vi "LOAD CELL FGV MAIN.vi"(7 "Enum":T2(ring), 8 "error in (no error)":errorcluster, 11 "main ref":T1) -> (0 "error IO":errorcluster)   [LabVIEW 2025]
uses:
  controls/LAB-IQ UI Data.ctl
  lib/hps_ft.dll
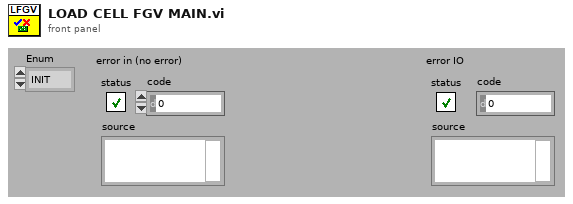
[diagram p1: front panel]
types:
  T1 = typedef "LAB-IQ UI Data.ctl" = cluster{"Main Home Screen":cluster{"GUI":refnum<vi>, "Platform Settings":refnum<vi>, "Configure":refnum<vi>, "Home":refnum<vi>, "EXIT":refnum<vi>, "service 2":refnum<vi>, "MainPage":refnum<vi>, "Analysis":refnum<vi>}, "Platform Settings":cluster{"mm/s  Surge":refnum<vi>, "Update Surge Speed":refnum<vi>, "Drive Error":refnum<vi>, "Disable Axis Jog Soft Limits":refnum<vi>, "mm/s  Sway":refnum<vi>, "Sway and Surge COM Status":refnum<vi>, "Heave COM Status":refnum<vi>, "Enable Platform":refnum<vi>, "Surge Forward Main":refnum<vi>, "Sway Right Main":refnum<vi>, "Sway Left Main":refnum<vi>, "Heave Down Main":refnum<vi>, "Heave Up main":refnum<vi>, "Update Sway Speed":refnum<vi>, "Update Heave Speed":refnum<vi>, "mm/s Heave":refnum<vi>, "mm/sec":refnum<vi>, "mm":refnum<vi>, "Surge Backward Main":refnum<vi>}, "Analysis Screen":cluster{"Analysis Home":refnum<vi>, "Surface Analysis":refnum<vi>, "Imaging":refnum<vi>, "Image Analysis":refnum<vi>, "Post Analysis":refnum<vi>}, "Config Screen":cluster{"Select Load Head":refnum<vi>, "Notes :":refnum<vi>, "FILE":refnum<vi>, "Sample ID :":refnum<vi>, "Operator ID :":refnum<vi>, "Operator Name :":refnum<vi>, "Auto":refnum<vi>}, "Motion Module":cluster{"zNL":refnum<vi>, "NL disp":refnum<vi>, "Rotary Tab":refnum<vi>, "Motion Direction:  3":refnum<vi>, "E.Velocity 2":refnum<vi>, "e.v/ssr 2":refnum<vi>, "Enter Fixed E.Velocity 2":refnum<vi>, "Enter Final SRR 2":refnum<vi>, "Enter initial SRR 2":refnum<vi>, "Enter Fixed SRR 2":refnum<vi>, "Enter the Final E.Velocity (m/s) 2":refnum<vi>, "Enter initial E.Velocity (m/s) 2":refnum<vi>, "Final Speed (RPM) 3":refnum<vi>, "Initial Speed (RPM) 2":refnum<vi>, "Enter the Final Velocity (m/s) 3":refnum<vi>, "Enter initial Velocity (m/s)  3":refnum<vi>, "Ramp Up 2":refnum<vi>, "TEST SELECTION":refnum<vi>, "SPEED SELECTION : ":refnum<vi>, "Angular Oscillation Set":refnum<vi>, "Traction":refnum<vi>, "Step Speed":refnum<vi>, "StepTable For Load-Speed":refnum<vi>, "StepTable For Speed":refnum<vi>, "Surge Forward MM":refnum<vi>, "Surge Backward MM":refnum<vi>, "M3 Image":refnum<vi>, "String 39":refnum<vi>, "Sway Left MM":refnum<vi>, "Sway Right MM":refnum<vi>, "Disable Axis Jog Soft Limits":refnum<vi>, "mm":refnum<vi>, "Heave Down MM":refnum<vi>, "Heave Up MM":refnum<vi>, "Wear Track Diameter (mm)":refnum<vi>, "Set WTD":refnum<vi>, "HomeScratch":refnum<vi>, "HomeRot":refnum<vi>, "PlaceModule":refnum<vi>, "Enter the Angle (Deg)":refnum<vi>, "Enter the Frequency (Hz)":refnum<vi>, "Motion Mode:":refnum<vi>, "LR Sway":refnum<vi>, "Rot Hor":refnum<vi>, "Scratch":refnum<vi>, "LR Cam":refnum<vi>, "MMBack":refnum<vi>, "MMNext":refnum<vi>, "Rot Ver":refnum<vi>, "Rotary Module Selection":refnum<vi>, "calculate rotary":refnum<vi>, "SPEED SELECTION : rotary":refnum<vi>, "Import 2":refnum<vi>, "Save 2":refnum<vi>, "File Path :  2":refnum<vi>, "String 45":refnum<vi>, "StepTable For Speed 3":refnum<vi>, "Enter the Speed(mm/sec)":refnum<vi>, "Enter the Speed(RPM)":refnum<vi>, "Enter Scratch Speed (mm/s):":refnum<vi>, "SwaySpeed Set":refnum<vi>, "Scartch Offset":refnum<vi>, "Motion type:":refnum<vi>, "HomeScratch 2":refnum<vi>, "Enter Scratch length (mm):":refnum<vi>, "Wear Track Diameter":refnum<vi>, "Rotary Speed Exced":refnum<vi>, "Scratch Mode":refnum<vi>, "No of Scratch":refnum<vi>}, "Environmental control":cluster{"Humidity  Status  3":refnum<vi>, "Low Temp  Status  2":refnum<vi>, "TK4 status 2":refnum<vi>, "Stage Temperature":refnum<vi>, "Sample Temperature":refnum<vi>, "Humidity (Amb)":refnum<vi>, "Clear List":refnum<vi>, "Add to list":refnum<vi>, "Wear":refnum<vi>, "Vibration":refnum<vi>, "Humidity (Chamber)":refnum<vi>, "Temperature (Chamber)":refnum<vi>, "ECR ":refnum<vi>, "Temperature (Amb)":refnum<vi>, "Microphone":refnum<vi>, "Acoustic Emission 3":refnum<vi>, "SNext":refnum<vi>, "APBack":refnum<vi>, "Enter the Temperature (°C):":refnum<vi>, "Enter the Stage \nTemperature (°C):":refnum<vi>, "Enter the Humidity (%Rh):":refnum<vi>, "Low Temp":refnum<vi>, "High Temp":refnum<vi>, "Humidity":refnum<vi>, "Sensors Picked":refnum<vi>}, "About Screen":cluster{"Password":refnum<vi>, "Home Service":refnum<vi>, "Advanced Setting":refnum<vi>, "About Tab":refnum<vi>, "ECR Port:":refnum<vi>, "Ramp Port:":refnum<vi>, "Installation/Replacement completed":refnum<vi>, "Loahead":refnum<vi>, "Heave and Surge COM Port:":refnum<vi>, "Sway COM Port:":refnum<vi>, "Temp Modbus:":refnum<vi>, "Humidity Port:":refnum<vi>, "Edit Gain Constants":refnum<vi>, "Save Gain Constants":refnum<vi>}, "Main Screen":cluster{"Main Screen Tab":refnum<vi>, "Angle and Frequency":refnum<vi>, "Stroke (mm)":refnum<vi>, "Angle (Deg)":refnum<vi>, "Main Speed Tab":refnum<vi>, "MTM MOTOR DISPLAY":refnum<vi>, "Disc Speed (m/sec)":refnum<vi>, "Ball Speed (m/sec)":refnum<vi>, "Disc Speed (RPM)":refnum<vi>, "Ball Speed (RPM)":refnum<vi>, "SPEED TAB":refnum<vi>, "Speed (m/sec)":refnum<vi>, "Set Speed (m/sec)":refnum<vi>, "Speed (RPM)":refnum<vi>, "Set Speed":refnum<vi>, "Time Tab":refnum<vi>, "Time ( HH:MM:SS ) 2":refnum<vi>, "Test Duration":refnum<vi>, "Test Duration 4":refnum<vi>, "TEST CYCLE":refnum<vi>, "TOTAL CYCLES":refnum<vi>, "Set Load (N)":refnum<vi>, "Temp Tabs":refnum<vi>, "Heater":refnum<vi>, "TK4 status":refnum<vi>, "ChamberTemp":refnum<vi>, "SetTmp":refnum<vi>, "Controller  Status":refnum<vi>, "ChamberTemp 2":refnum<vi>, "SetTmp 2":refnum<vi>, "Controller  Status 2":refnum<vi>, "ChamberTemp 3":refnum<vi>, "SetTmp 3":refnum<vi>, "Cooling":refnum<vi>, "Load Communication":refnum<vi>, "Ambient \nTemperature":refnum<vi>, "HumCOMStatus":refnum<vi>, "Ambient\n Humidity":refnum<vi>, "Freq (Hz)":refnum<vi>, "Load En":refnum<vi>, "NLt":refnum<vi>, "zNL 2":refnum<vi>, "Humidity On":refnum<vi>, "humidity disp":refnum<vi>, "Set Humidity":refnum<vi>, "NL disp 2":refnum<vi>, "Humidity On 2":refnum<vi>, "humidity disp 2":refnum<vi>, "Set Humidity 2":refnum<vi>, "NL disp 3":refnum<vi>, "AppLoadSeq scratch":refnum<vi>, "Stop Scratch":refnum<vi>, "ClrLog":refnum<vi>, "Trip Log":refnum<vi>, "STOP":refnum<vi>, "Start Test":refnum<vi>, "Test status":refnum<vi>, "AR Led":refnum<vi>, "Data":refnum<vi>, "Health":refnum<vi>, "Sway COM Status":refnum<vi>, "Heave COM Status":refnum<vi>, "Grp Tab":refnum<vi>, "Sub Graph":refnum<vi>, "SD (mm)":refnum<vi>, "Siliding distance Reset Graph":refnum<vi>, "SDGp":refnum<vi>, "Humidity Reset Graph":refnum<vi>, "HumrGp":refnum<vi>, "Acoustic Emission (mV)":refnum<vi>, "Aqucostic Reset Graph":refnum<vi>, "gACQUOS":refnum<vi>, "ECR RESET":refnum<vi>, "ECR":refnum<vi>, "Temperature Reset":refnum<vi>, "Acoustic Emission (mV) 2":refnum<vi>, "Aqucostic Reset Graph 2":refnum<vi>, "gACQUOS 2":refnum<vi>, "ECR RESET 2":refnum<vi>, "ECR 2":refnum<vi>, "Temperature Reset 2":refnum<vi>, "Temperature (deg c)":refnum<vi>, "Speed Reset Graph":refnum<vi>, "Speed Tab":refnum<vi>, "MTM DISC  SPEED":refnum<vi>, "MTM BALL SPEED":refnum<vi>, "speed mm/sec":refnum<vi>, "Hymidity":refnum<vi>, "Humidity Disable trip":refnum<vi>, "CoF Trip  2":refnum<vi>, "Depth Trip":refnum<vi>, "Weart Deapth":refnum<vi>, "Depth Reset Graph":refnum<vi>, "Weart":refnum<vi>, "Depthz":refnum<vi>, "Depth (µm)":refnum<vi>, "WearGp":refnum<vi>, "NL Trip 2":refnum<vi>, "Load pid":refnum<vi>, "Load Disable Trip":refnum<vi>, "Load Reset Graph":refnum<vi>, "NL Display 4":refnum<vi>, "Main Chart 3":refnum<vi>, "BACK":refnum<vi>, "Depth Trip 2":refnum<vi>, "COF TRIP ":refnum<vi>, "Friction Force (N)":refnum<vi>, "FF Reset Graph":refnum<vi>, "FF Disable Trip":refnum<vi>, "FF TRIP":refnum<vi>, "COF Disable Trip":refnum<vi>, "COF Reset Graph":refnum<vi>, "Start Test Temp":refnum<vi>, "zFF":refnum<vi>, "Friction Force (N) Graph":refnum<vi>, "Coefficient of Friction":refnum<vi>, "Scratch Start Test":refnum<vi>, "FF Tab":refnum<vi>, "Cyclic Friction Force (N)":refnum<vi>, "CZ FF":refnum<vi>, "Cyclic Friction Force (N) Graph":refnum<vi>, "Cyclic Coefficient of Friction":refnum<vi>, "Cyclic FF TRIP":refnum<vi>, "Cyclic FF Disable Trip":refnum<vi>, "cyclic COF Disable Trip":refnum<vi>, "cyclic COF TRIP":refnum<vi>, "cyclic COF Reset Graph":refnum<vi>, "Cyclic FF Reset Graph":refnum<vi>, "Test Trip":refnum<vi>, "Multi Scratch Pass":refnum<vi>, "Scratch Start Recording":refnum<vi>}, "Loading":cluster{"Indentation":refnum<vi>, "Reference Sample":refnum<vi>, "Load Cell Communication Slide":refnum<vi>, "com 3":refnum<vi>, "com":refnum<vi>, "DecaForce COM Status":refnum<vi>, "Update":refnum<vi>, "Clear 3":refnum<vi>, "seq":refnum<vi>, "Stribeck table":refnum<vi>, "Stribeck Table  For loading":refnum<vi>, "Loading Mode":refnum<vi>, "Enter the Final Load (N)":refnum<vi>, "Enter the CoF Trip":refnum<vi>, "Enter the Friction Force Trip":refnum<vi>, "Enter the Normal load Trip":refnum<vi>, "Enter the Load  (N)":refnum<vi>, "KiloForce":refnum<vi>, "DecaForce ":refnum<vi>, "MicroForce":refnum<vi>, "LHBack":refnum<vi>, "LHNext":refnum<vi>, "Enter the Loading Rate (N/min)":refnum<vi>, "Message":refnum<vi>, "Warning 2":refnum<vi>, "SSP 0.75":refnum<vi>, "SSP 0.5":refnum<vi>, "SSP 0.3":refnum<vi>, "Warning":refnum<vi>, "gui GIF":refnum<vi>, "Communication is established":refnum<vi>, "AppLoad 4":refnum<vi>, "Multipoint":refnum<vi>, "Load Selection":refnum<vi>}, "PID":cluster{"Ramp MulFac":refnum<vi>, "pulses LoadDiffRamp(2..10)":refnum<vi>, "PulseControlRamp(diff<=3N)":refnum<vi>, "SetLoadDeadband(%) Load(0-10N)":refnum<vi>, "PID gains out delay (microForce)":refnum<vi>, "Ramp":refnum<vi>, "Gain 2":refnum<vi>, "pulses LoadDiff(2..10)":refnum<vi>, "pulses LoadDiff(11..50)":refnum<vi>, "PulseControl(diff<=3N)":refnum<vi>, "SetLoadDeadband(%)  2":refnum<vi>, "Dummy Run":refnum<vi>, "Vertical load (N)":refnum<vi>, "AutoTune":refnum<vi>, "Offset 3 ":refnum<vi>, "apply load":refnum<vi>, "Offset  3":refnum<vi>, "apply load 2":refnum<vi>, "Enter ByPass Load":refnum<vi>, "reinit 3":refnum<vi>, "output range delay":refnum<vi>, "PID gains out delay":refnum<vi>, "Bypass Load":refnum<vi>, "pulsesSent":refnum<vi>, "pulses ":refnum<vi>, "actpid":refnum<vi>, "gFF Rot":refnum<vi>, "pulses LoadDiff(21..1000)":refnum<vi>, "Delay":refnum<vi>, "deadband":refnum<vi>}, "Config Parameters":cluster{"Tab Control 3":refnum<vi>, "Tab Control 19":refnum<vi>, "SAMPLES":refnum<vi>, "Re-initilaize":refnum<vi>, "Filter ON/OFF":refnum<vi>, "TracHomeSurgeOffsetCounts 10MM":refnum<vi>, "TracHomeSwayOffsetCounts 10MM":refnum<vi>, "Acoustic Emission:":refnum<vi>, "Apply Filter (FF)":refnum<vi>, "Filter% 2":refnum<vi>, "Apply Filter (Load)":refnum<vi>, "Filter% ":refnum<vi>, "Sway distance (mm)":refnum<vi>, "Surge distance (mm)":refnum<vi>, "DataSavingLoopDelay(ms)":refnum<vi>, "SAVE 2":refnum<vi>, "Enter Distance":refnum<vi>, "Sway Counts:":refnum<vi>, "Distance (mm): 3":refnum<vi>, "Surge Counts:":refnum<vi>, "Distance (mm): 2":refnum<vi>, "Distance (mm):":refnum<vi>, "Heave Counts:":refnum<vi>, "LRMHomeSurgeOffsetCounts":refnum<vi>, "LRMHomeSwayOffsetCounts":refnum<vi>, "TracHomeSurgeOffsetCounts 20MM":refnum<vi>, "TracHomeSwayOffsetCounts 20MM":refnum<vi>, "RotHomeSwayOffsetCounts":refnum<vi>, "RotHomeSurgeOffsetCounts":refnum<vi>, "Heave distance":refnum<vi>, "Zmm":refnum<vi>, "Heave Pulses/mm":refnum<vi>, "Surge Pulses/mm":refnum<vi>, "Sway Pulses/mm":refnum<vi>, "Heave Pitch":refnum<vi>, "Surge Pitch":refnum<vi>, "Sway Pitch":refnum<vi>, "Heave PPR":refnum<vi>, "Surge PPR":refnum<vi>, "Sway PPR":refnum<vi>, "Tab Control 5":refnum<vi>, "Tab Control 14":refnum<vi>, "Tab Control 26":refnum<vi>, "AE":refnum<vi>, "Heave Loop Delay":refnum<vi>, "Heave PID Speed":refnum<vi>, "Surge Jog Speed":refnum<vi>, "Heave Jog Speed":refnum<vi>, "Sway Loop Delay":refnum<vi>, "Sway PID Speed":refnum<vi>, "Sway Jog Speed":refnum<vi>, "DEPTH TRIP VALUE":refnum<vi>, "LOAD TRIP VALUE":refnum<vi>, "DEPTH TRIP   ENABLE":refnum<vi>, "LOAD TRIP  ENABLE":refnum<vi>, "CYCLIC FF TRIP VALUE":refnum<vi>, "FF TRIP VALUE":refnum<vi>, "CYCLIC CoF TRIP VALUE":refnum<vi>, "COF TRIP VALUE":refnum<vi>, "CYCLIC COF TRIP  ENABLE":refnum<vi>, "CYCLIC FF TRIP  ENABLE":refnum<vi>, "FF TRIP  ENABLE":refnum<vi>, "COF TRIP  ENABLE":refnum<vi>}, "Loading Com Port":cluster{"ClearAll":refnum<vi>, "Mz(Nm)":refnum<vi>, "My(Nm)":refnum<vi>, "Mx(Nm)":refnum<vi>, "Save Dwell":refnum<vi>, "Mx ":refnum<vi>, "My ":refnum<vi>, "Mz":refnum<vi>, "Fx(N)":refnum<vi>, "Fy(N)":refnum<vi>, "Fz(N)":refnum<vi>, "ZeroAll":refnum<vi>, "Acq Delay (ms)":refnum<vi>, "Burst Delay (ms)":refnum<vi>, "model":refnum<vi>, "SN":refnum<vi>, "FFx(N)":refnum<vi>, "Sensor IP":refnum<vi>, "Port":refnum<vi>, "FFy(N)":refnum<vi>, "Load(N)":refnum<vi>, "delete Handle":refnum<vi>, "Create Handle":refnum<vi>, "ft_data":refnum<vi>, "ft_range":refnum<vi>, "ft_data 2":refnum<vi>, "stop 6":refnum<vi>, "running_flag":refnum<vi>, "ft_udp_handle":refnum<vi>, "get-data-return":refnum<vi>, "get-range-return":refnum<vi>, "zero-return":refnum<vi>, "filter-return":refnum<vi>, "initial-return":refnum<vi>, "deleteHandle-result":refnum<vi>, "Load Cell Temp":refnum<vi>}, "Heave AND Surge":cluster{"SURGE POSE":refnum<vi>, "error out Read":refnum<vi>, "HEAVE POSE":refnum<vi>, "State":refnum<vi>, "Homed":refnum<vi>, "Sequence ID":refnum<vi>, "error out Write":refnum<vi>, "faultCode":refnum<vi>, "Ack ID":refnum<vi>, "SPEED":refnum<vi>, "Distance":refnum<vi>, "Mode Command":refnum<vi>, "Heave and Surge Read":refnum<vi>, "Read Heave Temp":refnum<vi>, "Spare 15":refnum<vi>, "Spare 14":refnum<vi>, "Spare 13":refnum<vi>, "Spare 12":refnum<vi>, "Spare 11":refnum<vi>, "Spare 10":refnum<vi>, "Spare 9":refnum<vi>, "Spare 8":refnum<vi>, "Spare 7":refnum<vi>, "Spare 6":refnum<vi>, "Spare 5":refnum<vi>, "Spare 4":refnum<vi>, "Spare 2":refnum<vi>, "Spare 1":refnum<vi>, "Node Id":refnum<vi>, "Spare 3":refnum<vi>, "SPARE 4":refnum<vi>, "SPARE 3":refnum<vi>, "SPARE 2":refnum<vi>, "SPARE 1":refnum<vi>, "fwMajor":refnum<vi>, "fwMinor":refnum<vi>, "Manual Write":refnum<vi>, "Heave and Surge Write":refnum<vi>}, "New PID LOGIC":cluster{"Fine Tune Zone":refnum<vi>, "PID SDelay":refnum<vi>, "Max_pos_limit":refnum<vi>, "Min_pos_limit":refnum<vi>, "i_limit":refnum<vi>, "pct_scale":refnum<vi>, "Deadband":refnum<vi>, "Kd":refnum<vi>, "Ki":refnum<vi>, "Kp":refnum<vi>, "Current Position":refnum<vi>, "Set Load":refnum<vi>, "Current Load":refnum<vi>, "Pulse delta":refnum<vi>, "Init Step":refnum<vi>, "Max Step Linit":refnum<vi>}, "SWAY ":cluster{"fwMajor":refnum<vi>, "Homed":refnum<vi>, "Rotary POSE":refnum<vi>, "State":refnum<vi>, "SWAY POSE":refnum<vi>, "Ack ID":refnum<vi>, "faultCode":refnum<vi>, "Node Id":refnum<vi>, "fwMinor":refnum<vi>, "Spare 6":refnum<vi>, "Spare 5":refnum<vi>, "Spare 4":refnum<vi>, "Spare 3":refnum<vi>, "Spare 2":refnum<vi>, "Spare 1":refnum<vi>, "Spare 7":refnum<vi>, "SPARE  5":refnum<vi>, "error out Write  SWAY ":refnum<vi>, "error out Read SWAY ":refnum<vi>, "Manual Write SWAY ":refnum<vi>, "SWAY WRITE":refnum<vi>, "SPARE  4":refnum<vi>, "SPARE  3":refnum<vi>, "SPARE 2":refnum<vi>, "SPARE 1":refnum<vi>, "Spare 15":refnum<vi>, "Spare 14":refnum<vi>, "Spare 13":refnum<vi>, "Spare 12":refnum<vi>, "Spare 11":refnum<vi>, "Spare 9":refnum<vi>, "Spare 8":refnum<vi>, "SPEED":refnum<vi>, "Distance":refnum<vi>, "Mode Command":refnum<vi>, "Sequence ID":refnum<vi>, "SWAY READ":refnum<vi>, "Spare 10":refnum<vi>, "Read SWAY Temp":refnum<vi>}, "Analysis Screen":cluster{"Analysis Home":refnum<vi>, "Refresh 2":refnum<vi>, "MEAN 4":refnum<vi>, "SD 4":refnum<vi>, "VARIANCE 4":refnum<vi>, "MEAN  3":refnum<vi>, "SD  3":refnum<vi>, "VARIANCE  3":refnum<vi>, "MEAN 2":refnum<vi>, "SD  2":refnum<vi>, "VARIANCE 2":refnum<vi>, "MEAN":refnum<vi>, "SD":refnum<vi>, "VARIANCE":refnum<vi>, "File 4 Discription":refnum<vi>, "OPEN 4":refnum<vi>, "File Name 4":refnum<vi>, "OPEN 3":refnum<vi>, "File 3 Discription":refnum<vi>, "File Name 3":refnum<vi>, "Y-AXIS":refnum<vi>, "X-AXIS":refnum<vi>, "XY Graph":refnum<vi>, "File Name 2":refnum<vi>, "File Name 1":refnum<vi>, "OPEN 2":refnum<vi>, "OPEN 1":refnum<vi>, "File 1 Discription ":refnum<vi>, "File 2 Discription":refnum<vi>, "Export":refnum<vi>, "File Format":refnum<vi>}}
  T2 = enum16{"INIT", "SETLOWPASSFILTER", "SETZERO", "GETSENSORINFO", "GETRANGE", "ZEROALL", "READDATA", "UNINITIAL", "DELETEHANDLE"}
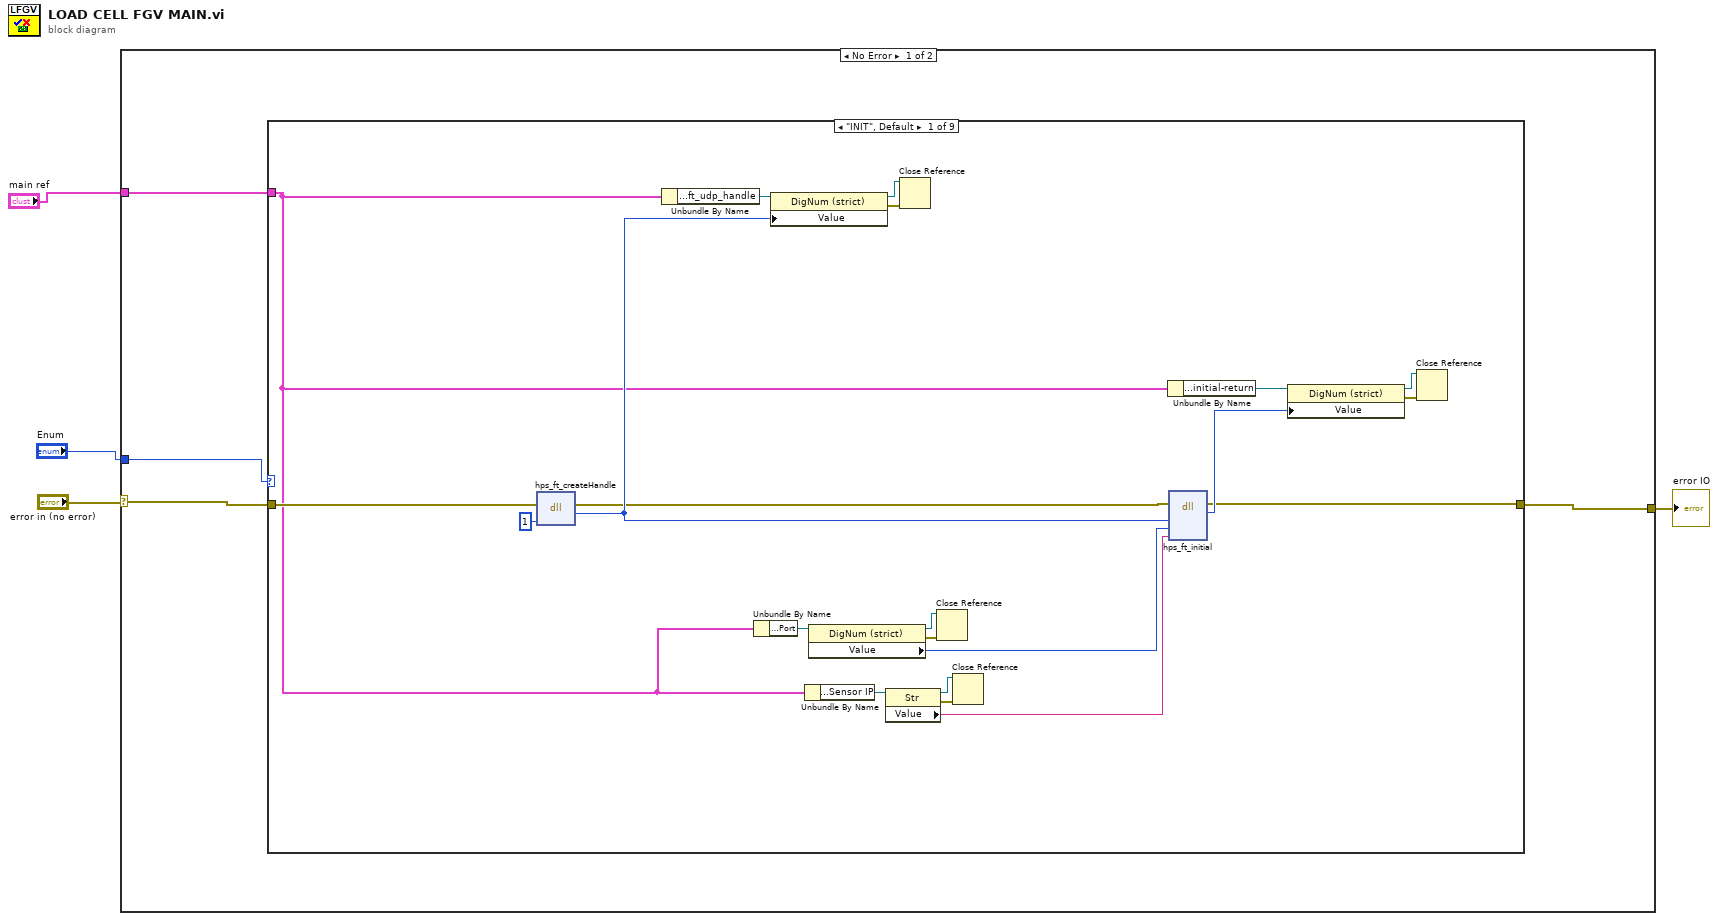
[diagram p0: block diagram]
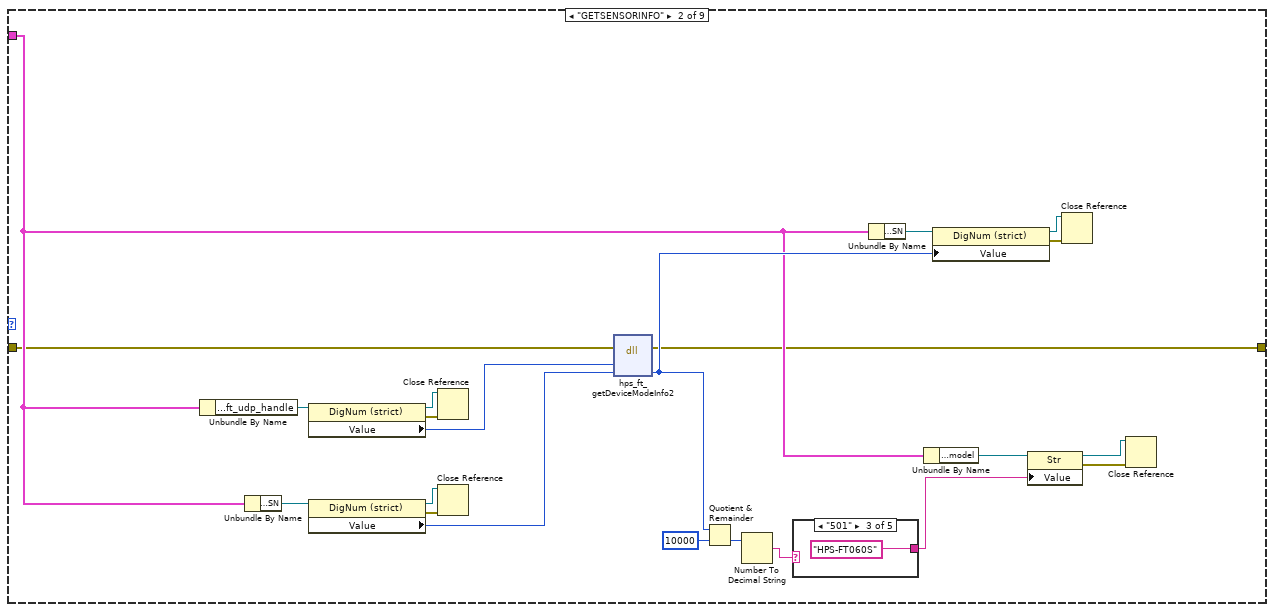
[diagram p2: hidden frame]
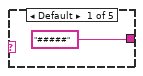
[diagram p3: hidden frame]
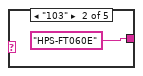
[diagram p4: hidden frame]
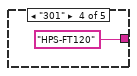
[diagram p5: hidden frame]
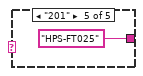
[diagram p6: hidden frame]
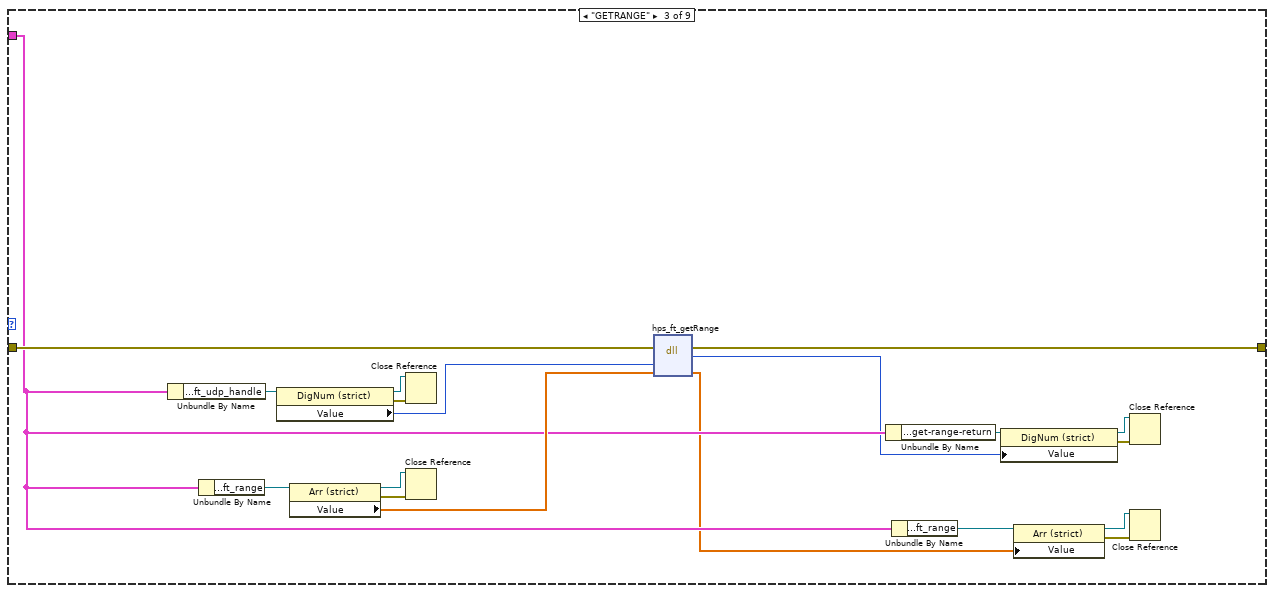
[diagram p7: hidden frame]
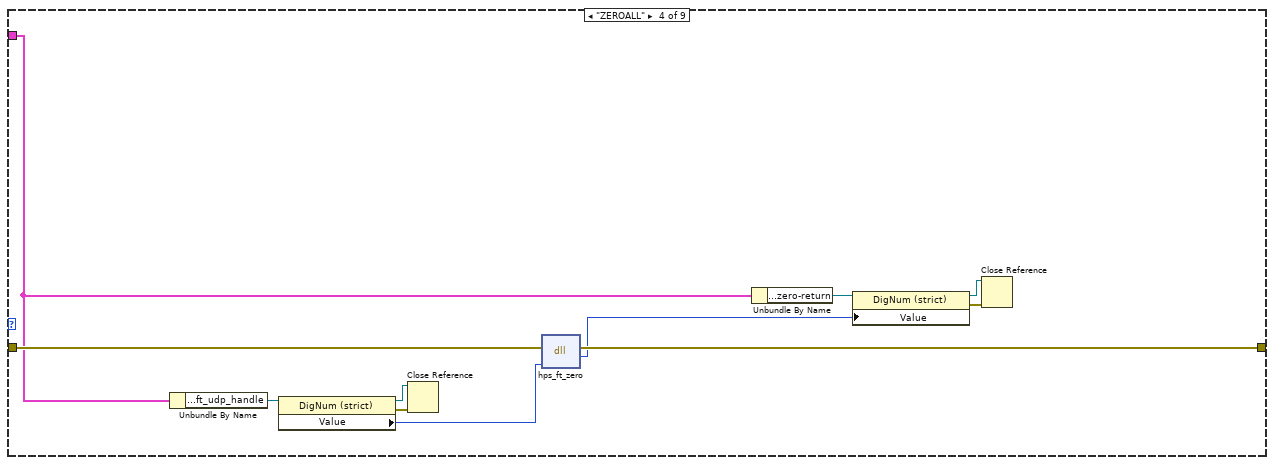
[diagram p8: hidden frame]
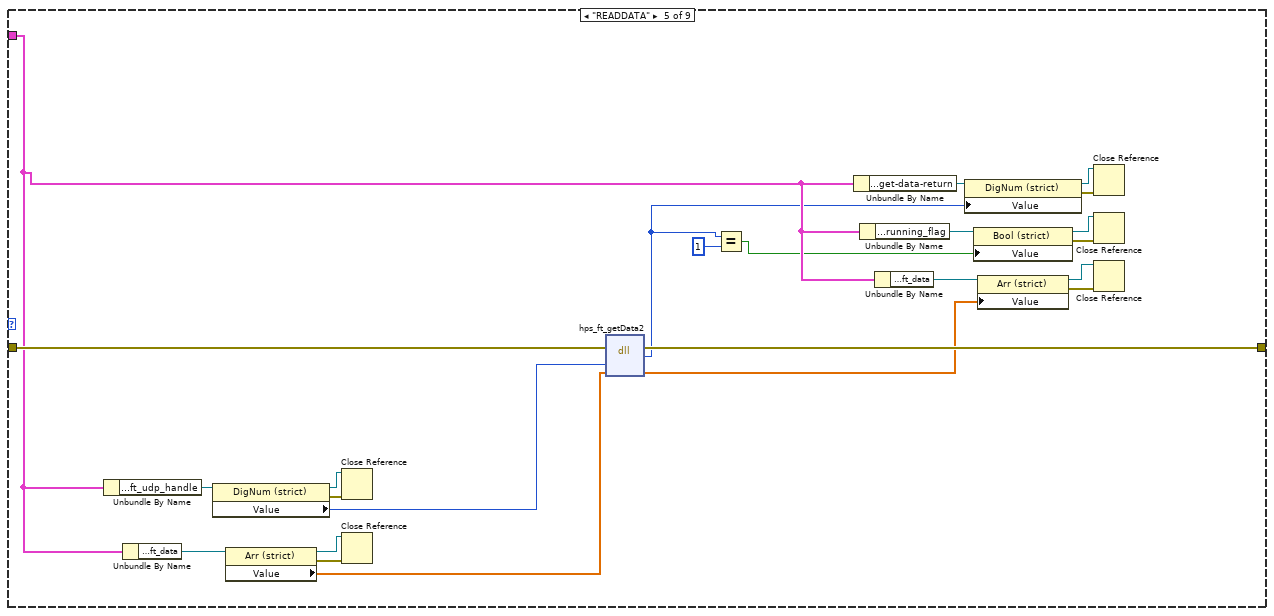
[diagram p9: hidden frame]
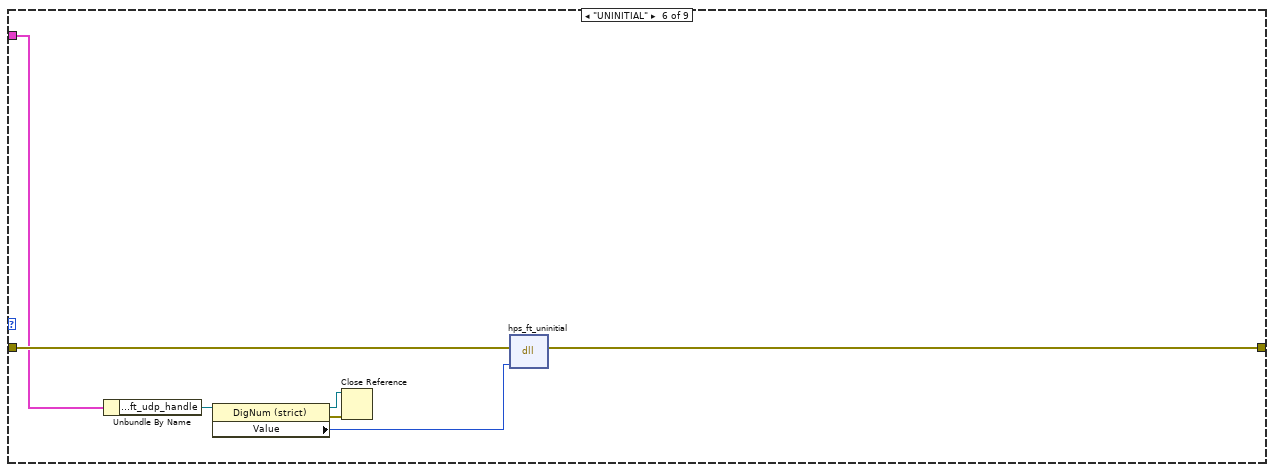
[diagram p10: hidden frame]
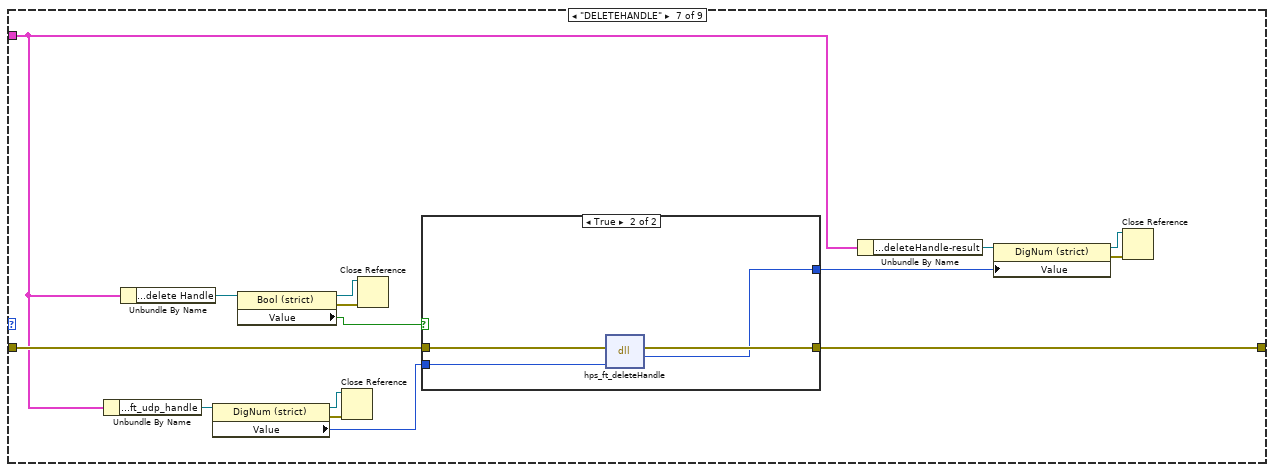
[diagram p11: hidden frame]
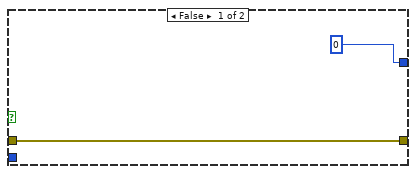
[diagram p12: hidden frame]
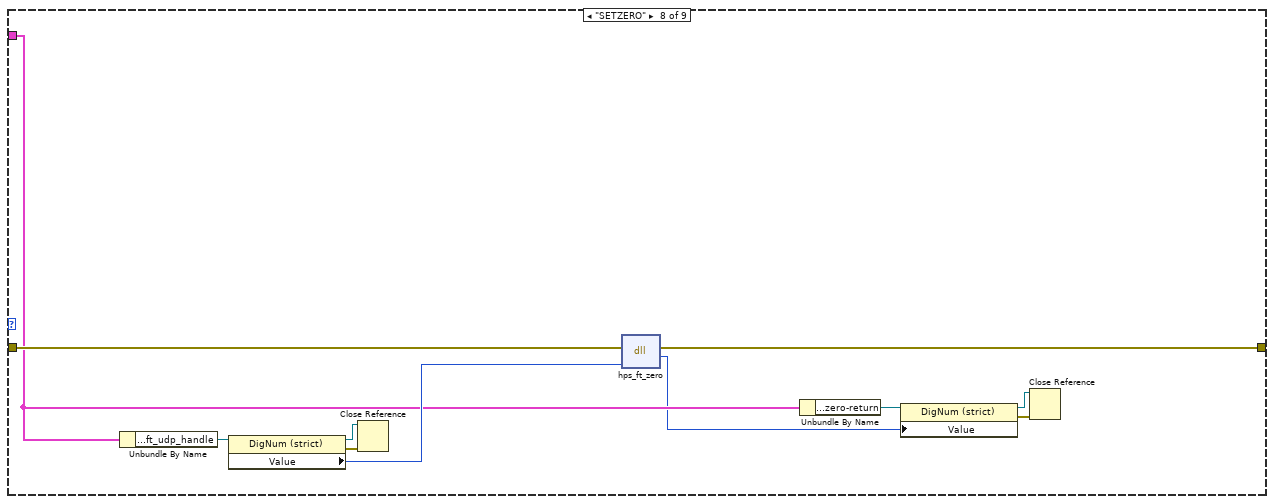
[diagram p13: hidden frame]
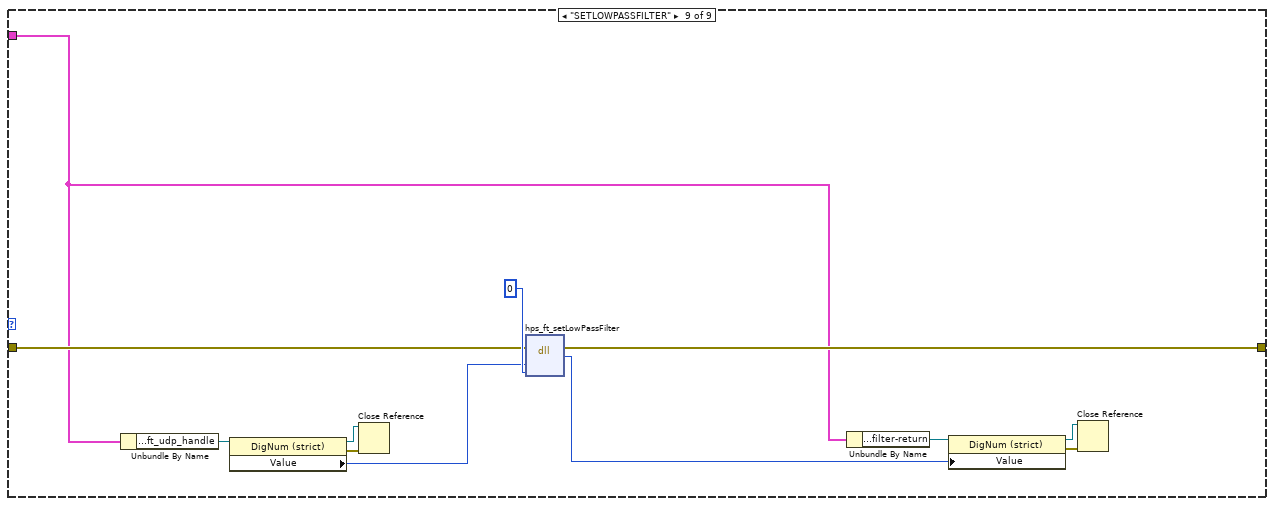
[diagram p14: hidden frame]
diagram:
  n1 = case shown="No Error" "error in (no error)" {
    selector: "error in (no error)" -> [w8 _]
    tunnel: [w7 _] -> w3
    tunnel: "Enum" -> [w6 _]
    tunnel: "main ref" -> [w5 _]
    frame No Error {
      n2 = case shown="\"INIT\", Default" w6 {
        tunnel: w8 -> [w16 w31 w75 w86 w109 w117 w132 w149 w160]
        tunnel: [w9 w30 w74 w85 w108 w116 w131 w139 w159] -> w7
        tunnel: w5 -> [w11 w33 w59 w77 w91 w111 w119 w141 w151]
        frame "INIT", Default {
          n3 = dll-call lib="D:/LAB-IQ 150/lib/hps_ft.dll" fn="hps_ft_createHandle"(error in=w16, "1(UDP)"=1) -> (error out=w15:errorcluster, "return type"=w25:i32)  [unwired: 3 in, 1 out]
          n4 = Unbundle By Name(w11) -> ("Loading Com Port.ft_udp_handle"=w26:refnum<vi>)
          n5 = Unbundle By Name(w11) -> ("Loading Com Port.Port"=w20:refnum<vi>)
          n6 = property class="DigNum (strict)"(reference=w26, "Value"=w25) -> (reference out=w28:refnum<vi>, error out=w27:errorcluster)  [unwired: 1 in]
          n7 = Unbundle By Name(w11) -> ("Loading Com Port.Sensor IP"=w24:refnum<vi>)
          n8 = property class="DigNum (strict)"(reference=w20) -> (reference out=w19:refnum<vi>, error out=w21:errorcluster, "Value"=w18:i32)  [unwired: 1 in]
          n9 = property class="Str"(reference=w24) -> (reference out=w22:refnum<vi>, error out=w23:errorcluster, "Value"=w17:string)  [unwired: 1 in]
          n10 = Close Reference(reference=w28, error in (no error)=w27) -> ()  [unwired: 1 out]
          n11 = Close Reference(reference=w19, error in (no error)=w21) -> ()  [unwired: 1 out]
          n12 = Close Reference(reference=w22, error in (no error)=w23) -> ()  [unwired: 1 out]
          n13 = Unbundle By Name(w11) -> ("Loading Com Port.initial-return"=w14:refnum<vi>)
          n14 = dll-call lib="D:/LAB-IQ 150/lib/hps_ft.dll" fn="hps_ft_initial"(error in=w15, "handle"=w25, "port"=w18, "IP"=w17) -> (error out=w9:errorcluster, "return type"=w10:i32)  [unwired: 5 in, 1 out]
          n15 = property class="DigNum (strict)"(reference=w14, "Value"=w10) -> (reference out=w12:refnum<vi>, error out=w13:errorcluster)  [unwired: 1 in]
          n16 = Close Reference(reference=w12, error in (no error)=w13) -> ()  [unwired: 1 out]
        }
        frame "GETSENSORINFO" {
          n17 = Unbundle By Name(w33) -> ("Loading Com Port.ft_udp_handle"=w46:refnum<vi>)
          n18 = Unbundle By Name(w33) -> ("Loading Com Port.SN"=w43:refnum<vi>)
          n19 = property class="DigNum (strict)"(reference=w46) -> (reference out=w48:refnum<vi>, error out=w47:errorcluster, "Value"=w42:i32)  [unwired: 1 in]
          n20 = property class="DigNum (strict)"(reference=w43) -> (reference out=w45:refnum<vi>, error out=w44:errorcluster, "Value"=w41:i32)  [unwired: 1 in]
          n21 = Close Reference(reference=w48, error in (no error)=w47) -> ()  [unwired: 1 out]
          n22 = Close Reference(reference=w45, error in (no error)=w44) -> ()  [unwired: 1 out]
          n23 = dll-call lib="D:/LAB-IQ 150/lib/hps_ft.dll" fn="hps_ft_getDeviceModeInfo2"(error in=w31, "handle"=w42, "sensor_info"=w41) -> (error out=w30:errorcluster, "sensor_info"=w37:i32)  [unwired: 4 in, 1 out]
          n24 = Quotient & Remainder(x=w37, y=10000) -> (floor(x/y)=w51:i32)  [unwired: 1 out]
          n25 = Number To Decimal String(number=w51) -> (decimal integer string=w49:string)  [unwired: 1 in]
          n26 = case shown="\"501\"" w49 {
            tunnel: ["#####" "HPS-FT060E" "HPS-FT060S" "HPS-FT120" "HPS-FT025"] -> w32
            frame Default {
            }
            frame "103" {
            }
            frame "501" {
            }
            frame "301" {
            }
            frame "201" {
            }
          }
          n27 = Unbundle By Name(w33) -> ("Loading Com Port.SN"=w40:refnum<vi>)
          n28 = Unbundle By Name(w33) -> ("Loading Com Port.model"=w34:refnum<vi>)
          n29 = property class="DigNum (strict)"(reference=w40, "Value"=w37) -> (reference out=w38:refnum<vi>, error out=w39:errorcluster)  [unwired: 1 in]
          n30 = property class="Str"(reference=w34, "Value"=w32) -> (reference out=w36:refnum<vi>, error out=w35:errorcluster)  [unwired: 1 in]
          n31 = Close Reference(reference=w38, error in (no error)=w39) -> ()  [unwired: 1 out]
          n32 = Close Reference(reference=w36, error in (no error)=w35) -> ()  [unwired: 1 out]
        }
        frame "GETRANGE" {
          n33 = Unbundle By Name(w59) -> ("Loading Com Port.ft_udp_handle"=w71:refnum<vi>)
          n34 = Unbundle By Name(w59) -> ("Loading Com Port.ft_range"=w68:refnum<vi>)
          n35 = property class="DigNum (strict)"(reference=w71) -> (reference out=w73:refnum<vi>, error out=w72:errorcluster, "Value"=w67:i32)  [unwired: 1 in]
          n36 = property class="Arr (strict)"(reference=w68) -> (reference out=w70:refnum<vi>, error out=w69:errorcluster, "Value"=w66:dbl[])  [unwired: 1 in]
          n37 = Close Reference(reference=w73, error in (no error)=w72) -> ()  [unwired: 1 out]
          n38 = Close Reference(reference=w70, error in (no error)=w69) -> ()  [unwired: 1 out]
          n39 = dll-call lib="D:/LAB-IQ 150/lib/hps_ft.dll" fn="hps_ft_getRange"(error in=w75, "handle"=w67, "fi_data"=w66) -> (error out=w74:errorcluster, "return type"=w57:i32, "fi_data"=w58:dbl[])  [unwired: 3 in, 1 out]
          n40 = Unbundle By Name(w59) -> ("Loading Com Port.get-range-return"=w63:refnum<vi>)
          n41 = Unbundle By Name(w59) -> ("Loading Com Port.ft_range"=w60:refnum<vi>)
          n42 = property class="DigNum (strict)"(reference=w63, "Value"=w57) -> (reference out=w65:refnum<vi>, error out=w64:errorcluster)  [unwired: 1 in]
          n43 = property class="Arr (strict)"(reference=w60, "Value"=w58) -> (reference out=w62:refnum<vi>, error out=w61:errorcluster)  [unwired: 1 in]
          n44 = Close Reference(reference=w65, error in (no error)=w64) -> ()  [unwired: 1 out]
          n45 = Close Reference(reference=w62, error in (no error)=w61) -> ()  [unwired: 1 out]
        }
        frame "ZEROALL" {
          n46 = Unbundle By Name(w77) -> ("Loading Com Port.ft_udp_handle"=w82:refnum<vi>)
          n47 = property class="DigNum (strict)"(reference=w82) -> (reference out=w84:refnum<vi>, error out=w83:errorcluster, "Value"=w81:i32)  [unwired: 1 in]
          n48 = Close Reference(reference=w84, error in (no error)=w83) -> ()  [unwired: 1 out]
          n49 = dll-call lib="D:/LAB-IQ 150/lib/hps_ft.dll" fn="hps_ft_zero"(error in=w86, "handle"=w81) -> (error out=w85:errorcluster, "return type"=w76:i32)  [unwired: 3 in, 1 out]
          n50 = Unbundle By Name(w77) -> ("Loading Com Port.zero-return"=w78:refnum<vi>)
          n51 = property class="DigNum (strict)"(reference=w78, "Value"=w76) -> (reference out=w80:refnum<vi>, error out=w79:errorcluster)  [unwired: 1 in]
          n52 = Close Reference(reference=w80, error in (no error)=w79) -> ()  [unwired: 1 out]
        }
        frame "READDATA" {
          n53 = Unbundle By Name(w91) -> ("Loading Com Port.ft_udp_handle"=w105:refnum<vi>)
          n54 = Unbundle By Name(w91) -> ("Loading Com Port.ft_data"=w104:refnum<vi>)
          n55 = property class="DigNum (strict)"(reference=w105) -> (reference out=w107:refnum<vi>, error out=w106:errorcluster, "Value"=w101:i32)  [unwired: 1 in]
          n56 = property class="Arr (strict)"(reference=w104) -> (reference out=w102:refnum<vi>, error out=w103:errorcluster, "Value"=w100:dbl[])  [unwired: 1 in]
          n57 = Close Reference(reference=w107, error in (no error)=w106) -> ()  [unwired: 1 out]
          n58 = Close Reference(reference=w102, error in (no error)=w103) -> ()  [unwired: 1 out]
          n59 = dll-call lib="D:/LAB-IQ 150/lib/hps_ft.dll" fn="hps_ft_getData2"(error in=w109, "handle"=w101, "fi_data"=w100) -> (error out=w108:errorcluster, "return type"=w90:i32, "fi_data"=w88:dbl[])  [unwired: 3 in, 1 out]
          n60 = Equal?(x=w90, y=1) -> (x = y?=w89:bool)
          n61 = Unbundle By Name(w91) -> ("Loading Com Port.get-data-return"=w99:refnum<vi>)
          n62 = Unbundle By Name(w91) -> ("Loading Com Port.running_flag"=w94:refnum<vi>)
          n63 = Unbundle By Name(w91) -> ("Loading Com Port.ft_data"=w93:refnum<vi>)
          n64 = property class="DigNum (strict)"(reference=w99, "Value"=w90) -> (reference out=w97:refnum<vi>, error out=w98:errorcluster)  [unwired: 1 in]
          n65 = property class="Bool (strict)"(reference=w94, "Value"=w89) -> (reference out=w96:refnum<vi>, error out=w95:errorcluster)  [unwired: 1 in]
          n66 = property class="Arr (strict)"(reference=w93, "Value"=w88) -> (reference out=w87:refnum<vi>, error out=w92:errorcluster)  [unwired: 1 in]
          n67 = Close Reference(reference=w97, error in (no error)=w98) -> ()  [unwired: 1 out]
          n68 = Close Reference(reference=w96, error in (no error)=w95) -> ()  [unwired: 1 out]
          n69 = Close Reference(reference=w87, error in (no error)=w92) -> ()  [unwired: 1 out]
        }
        frame "UNINITIAL" {
          n70 = Unbundle By Name(w111) -> ("Loading Com Port.ft_udp_handle"=w113:refnum<vi>)
          n71 = property class="DigNum (strict)"(reference=w113) -> (reference out=w115:refnum<vi>, error out=w114:errorcluster, "Value"=w112:i32)  [unwired: 1 in]
          n72 = Close Reference(reference=w115, error in (no error)=w114) -> ()  [unwired: 1 out]
          n73 = dll-call lib="D:/LAB-IQ 150/lib/hps_ft.dll" fn="hps_ft_uninitial"(error in=w117, "handle"=w112) -> (error out=w116:errorcluster)  [unwired: 4 in, 1 out]
        }
        frame "DELETEHANDLE" {
          n74 = Unbundle By Name(w119) -> ("Loading Com Port.ft_udp_handle"=w128:refnum<vi>)
          n75 = Unbundle By Name(w119) -> ("Loading Com Port.delete Handle"=w126:refnum<vi>)
          n76 = property class="DigNum (strict)"(reference=w128) -> (reference out=w130:refnum<vi>, error out=w129:errorcluster, "Value"=w127:i32)  [unwired: 1 in]
          n77 = property class="Bool (strict)"(reference=w126) -> (reference out=w124:refnum<vi>, error out=w125:errorcluster, "Value"=w123:bool)  [unwired: 1 in]
          n78 = Close Reference(reference=w130, error in (no error)=w129) -> ()  [unwired: 1 out]
          n79 = Close Reference(reference=w124, error in (no error)=w125) -> ()  [unwired: 1 out]
          n80 = case shown="True" w123 {
            tunnel: w127 -> [_ w138]
            tunnel: w132 -> [w134 w137]
            tunnel: [w134 w136] -> w131
            tunnel: [0 w135] -> w118
            frame False {
            }
            frame True {
              n81 = dll-call lib="D:/LAB-IQ 150/lib/hps_ft.dll" fn="hps_ft_deleteHandle"(error in=w137, "handle"=w138) -> (error out=w136:errorcluster, "return type"=w135:i32)  [unwired: 3 in, 1 out]
            }
          }
          n82 = Unbundle By Name(w119) -> ("Loading Com Port.deleteHandle-result"=w122:refnum<vi>)
          n83 = property class="DigNum (strict)"(reference=w122, "Value"=w118) -> (reference out=w120:refnum<vi>, error out=w121:errorcluster)  [unwired: 1 in]
          n84 = Close Reference(reference=w120, error in (no error)=w121) -> ()  [unwired: 1 out]
        }
        frame "SETZERO" {
          n85 = Unbundle By Name(w141) -> ("Loading Com Port.ft_udp_handle"=w148:refnum<vi>)
          n86 = property class="DigNum (strict)"(reference=w148) -> (reference out=w146:refnum<vi>, error out=w147:errorcluster, "Value"=w145:i32)  [unwired: 1 in]
          n87 = Close Reference(reference=w146, error in (no error)=w147) -> ()  [unwired: 1 out]
          n88 = dll-call lib="D:/LAB-IQ 150/lib/hps_ft.dll" fn="hps_ft_zero"(error in=w149, "handle"=w145) -> (error out=w139:errorcluster, "return type"=w140:i32)  [unwired: 3 in, 1 out]
          n89 = Unbundle By Name(w141) -> ("Loading Com Port.zero-return"=w144:refnum<vi>)
          n90 = property class="DigNum (strict)"(reference=w144, "Value"=w140) -> (reference out=w142:refnum<vi>, error out=w143:errorcluster)  [unwired: 1 in]
          n91 = Close Reference(reference=w142, error in (no error)=w143) -> ()  [unwired: 1 out]
        }
        frame "SETLOWPASSFILTER" {
          n92 = Unbundle By Name(w151) -> ("Loading Com Port.ft_udp_handle"=w158:refnum<vi>)
          n93 = property class="DigNum (strict)"(reference=w158) -> (reference out=w155:refnum<vi>, error out=w157:errorcluster, "Value"=w156:i32)  [unwired: 1 in]
          n94 = Close Reference(reference=w155, error in (no error)=w157) -> ()  [unwired: 1 out]
          n95 = dll-call lib="D:/LAB-IQ 150/lib/hps_ft.dll" fn="hps_ft_setLowPassFilter"(error in=w160, "handle"=w156, "level"=0) -> (error out=w159:errorcluster, "return type"=w150:i32)  [unwired: 4 in, 1 out]
          n96 = Unbundle By Name(w151) -> ("Loading Com Port.filter-return"=w154:refnum<vi>)
          n97 = property class="DigNum (strict)"(reference=w154, "Value"=w150) -> (reference out=w152:refnum<vi>, error out=w153:errorcluster)  [unwired: 1 in]
          n98 = Close Reference(reference=w152, error in (no error)=w153) -> ()  [unwired: 1 out]
        }
      }
    }
    frame Error {
    }
  }
  "error IO" <- w3
